vi "Do.vi"(8 "error in (no error)":errorcluster, 10 "Actor in":refnum<class "Actor.lvclass">, 11 "Update PV Msg":refnum<class "Update PV Msg.lvclass">) -> (0 "error out":errorcluster, 2 "Actor out":refnum<class "Actor.lvclass">)   [LabVIEW 2013, in "CS++FgenGui.lvlib" / "Update PV Msg.lvclass"]
doc: "This VI delivers the message to the actor by calling the appropriate method(s) on the actor."
uses:
  Update PV Msg.lvclass
  <vilib>/ActorFramework/Actor/Actor.lvclass
  CS++FgenGui/CS++FgenGui.lvclass
  Core/Actors/CS++PVMonitor Messages/CS++PVUpdate Msg/CS++PVUpdate Msg.lvclass/CS++PVUpdate Msg.ctl
  Core/Classes/CS++ProcessVariables/ProcessVariable/PV.lvclass
  Core/Actors/CS++PVMonitor Messages/CS++PVUpdate Msg/CS++PVUpdate Msg.lvclass
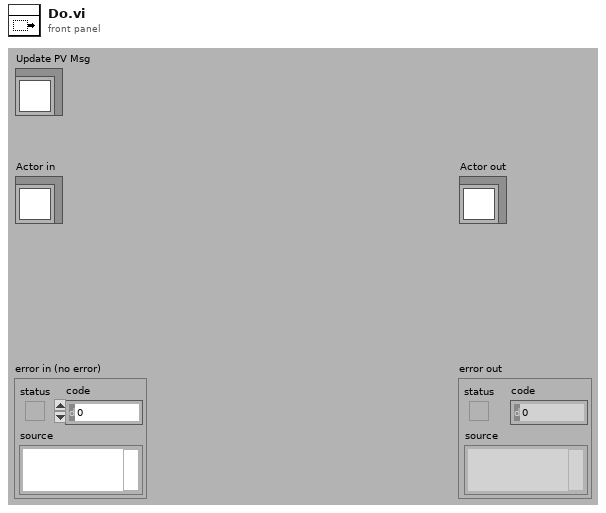
[diagram p1: front panel]
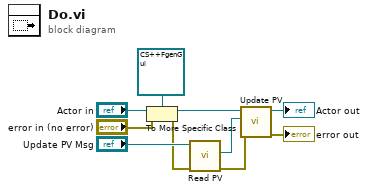
[diagram p0: block diagram]
diagram:
  n1 = To More Specific Class(target class=refnum<class "CS++FgenGui.lvclass"> refnum ("CS++FgenGui.lvlib:CS++FgenGui.lvclass"), reference="Actor in", error in="error in (no error)") -> (specific class reference=w5:refnum<class "CS++FgenGui.lvclass">, error out=w3:errorcluster)
  n2 = call "Read PV.vi"("error in (no error)"=w3, "CS++PVUpdate Msg in"="Update PV Msg") -> ("error out"=w2:errorcluster, "PV"=w1:refnum<class "PV.lvclass">)  [unwired: 7 in, 1 out]
  n3 = call "Update PV.vi"("error in (no error)"=w2, "PV"=w1, "CS++FgenGui in"=w5) -> ("error out"=→"error out":errorcluster, "CS++FgenGui out"=→"Actor out":refnum<class "CS++FgenGui.lvclass">)  [unwired: 7 in]
